vi "IsWindow.vi"(8 "error in (no error)":errorcluster, 11 "hWnd (NULL)":T1) -> (0 "error out":errorcluster, 2 "Is Window?":bool, 3 "dup hWnd":T1)   [LabVIEW 2011]
uses:
  hWnd.ctl
  user32.dll
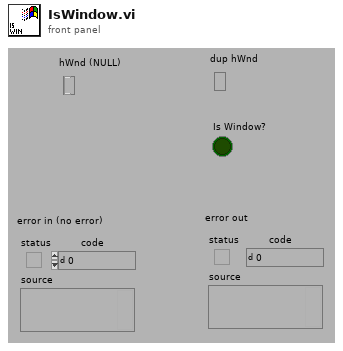
[diagram p1: front panel]
types:
  T1 = typedef "hWnd.ctl" = refnum<k1>
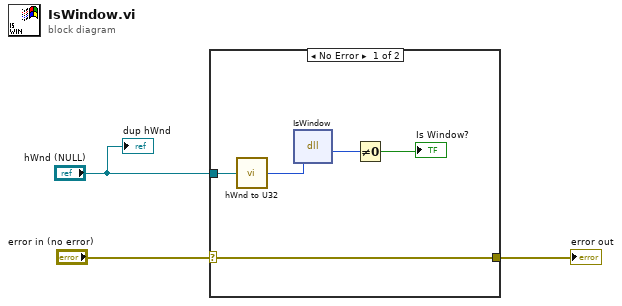
[diagram p0: block diagram]
diagram:
  n1 = case shown="No Error" "error in (no error)" {
    selector: "error in (no error)" -> [w4 w9]
    tunnel: "hWnd (NULL)" -> [w6 _]
    tunnel: [w4 w9] -> w3
    frame No Error {
      n2 = call "hWnd to U32.vi"("hWnd"=w6) -> ("hWnd"=w5:u32)  [unwired: 4 out]
      n3 = dll-call lib="User32.dll" fn="IsWindow"("hWnd"=w5) -> ("IsWindow?"=w8:i32)  [unwired: 4 in, 2 out]
      n4 = Not Equal To 0?(x=w8) -> (x != 0?=→"Is Window?":bool)
    }
    frame Error {
    }
  }
  "error out" <- w3
  "dup hWnd" <- "hWnd (NULL)"
